vi "ScrollbarMinMax.vi"(2 "Scrollbar Min (V) 2":dbl=-10.0 min=-10.0 max=10.0, 3 "Scrollbar Max (V) 2":dbl=10.0 min=-10.0 max=10.0, 4 "Upper/Lower":bool) -> (0 "New Scrollbar Min":dbl, 1 "New Scrollbar Max":dbl)   [LabVIEW 2017]
panel:
  out "Inbetween":dbl
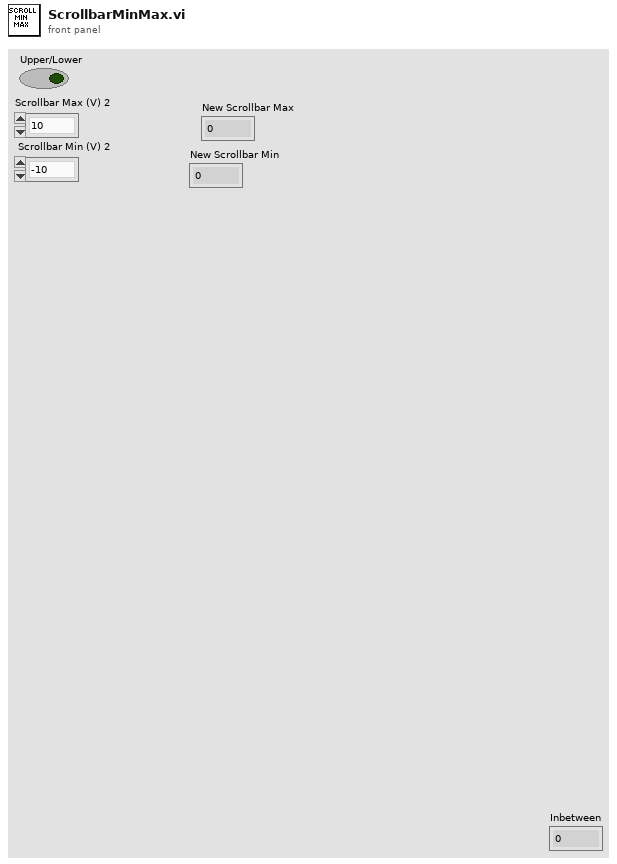
[diagram p1: front panel]
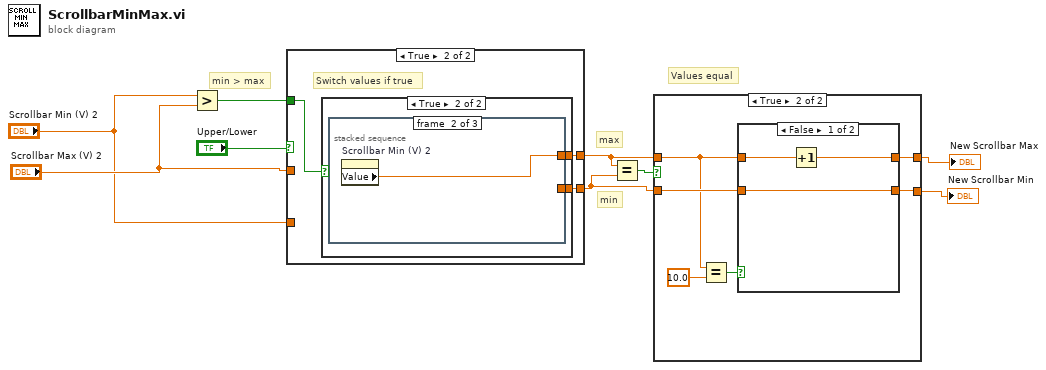
[diagram p0: block diagram]
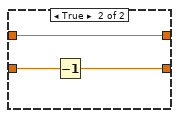
[diagram p3: hidden frame]
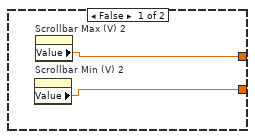
[diagram p5: hidden frame]
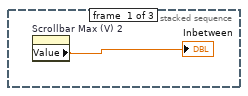
[diagram p6: hidden frame]
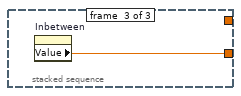
[diagram p7: hidden frame]
diagram:
  # "Values equal"
  # "min"
  # "max"
  # "min > max"
  n1 = Greater?(x="Scrollbar Min (V) 2", y="Scrollbar Max (V) 2") -> (0:w8:bool)
  n2 = case shown="True" "Upper/Lower" {
    tunnel: w8 -> [_ w14]
    tunnel: [w10 w13] -> w3
    tunnel: [w11 w12] -> w4
    tunnel: "Scrollbar Max (V) 2" -> [w11 _]
    tunnel: "Scrollbar Min (V) 2" -> [w10 _]
    frame False {
      # "Switch values if true"
    }
    frame True {
      # "Switch values if true"
      n3 = case shown="True" w14 {
        tunnel: [w15 w18] -> w13
        tunnel: [w16 w17] -> w12
        frame False {
          n4 = property on="Scrollbar Min (V) 2" class="DigNum (strict)"() -> ("Value"=w15:dbl)  [unwired: 2 in, 2 out]
          n5 = property on="Scrollbar Max (V) 2" class="DigNum (strict)"() -> ("Value"=w16:dbl)  [unwired: 2 in, 2 out]
        }
        frame True {
          n6 = stacked-sequence {
            tunnel: [_ _ w21] -> w18
            tunnel: [_ w20 _] -> w17
            frame #0 {
              n7 = property on="Scrollbar Max (V) 2" class="DigNum (strict)"() -> ("Value"=→"Inbetween":dbl)  [unwired: 2 in, 2 out]
            }
            frame #1 {
              n8 = property on="Scrollbar Min (V) 2" class="DigNum (strict)"() -> ("Value"=w20:dbl)  [unwired: 2 in, 2 out]
            }
            frame #2 {
              n9 = property on="Inbetween" class="DigNum (strict)"() -> ("Value"=w21:dbl)  [unwired: 2 in, 2 out]
            }
          }
        }
      }
    }
  }
  n10 = Equal?(x=w4, y=w3) -> (x = y?=w5:bool)
  n11 = case shown="True" w5 {
    tunnel: w4 -> [w23 w26]
    tunnel: w3 -> [w22 w29]
    tunnel: [w22 w25] -> w1
    tunnel: [w23 w24] -> w2
    frame False {
    }
    frame True {
      n12 = Equal?(x=w26, y=10.0) -> (x = y?=w28:bool)
      n13 = case shown="False" w28 {
        tunnel: w26 -> [w32 w34]
        tunnel: w29 -> [w31 w35]
        tunnel: [w31 w33] -> w25
        tunnel: [w30 w34] -> w24
        frame False {
          n14 = Increment(x=w32) -> (x+1=w30:dbl)
        }
        frame True {
          n15 = Decrement(x=w35) -> (x-1=w33:dbl)
        }
      }
    }
  }
  "New Scrollbar Min" <- w1
  "New Scrollbar Max" <- w2
